vi "Replicate Graph.vi"() -> ()   [LabVIEW 2020, in "Uno.lvclass"]
uses:
  Uno.lvclass
  <vilib>/Analysis/1siggen.llb/Ramp Pattern by Delta.vi
  <vilib>/Analysis/NI_AALBase.lvlib
panel:
  out "Waveform Graph":dbl[][](graph)
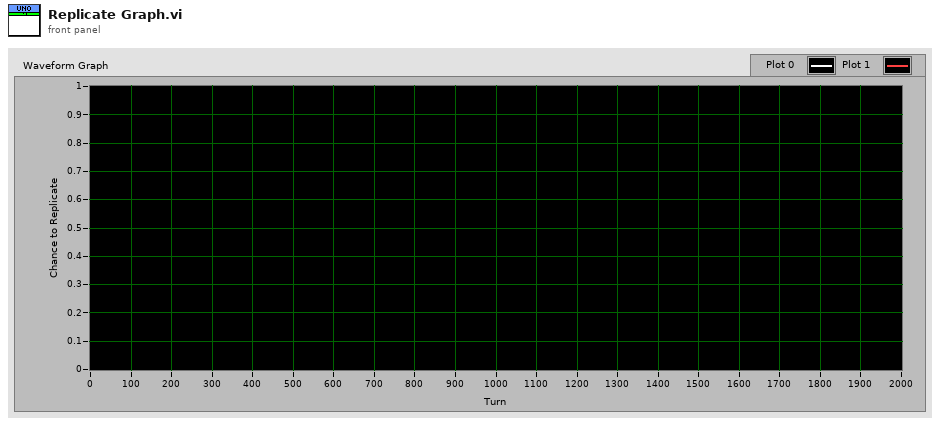
[diagram p1: front panel]
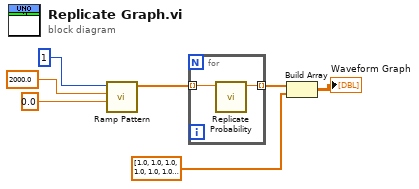
[diagram p0: block diagram]
diagram:
  n1 = call-poly <vilib>:"Ramp Pattern.vi"("start"=0.0, "end"=2000.0, "delta"=1 ("samples")) -> ("Ramp Pattern"=w4:dbl[])  [unwired: 6 in, 2 out]
  n2 = for {
    tunnel: w4 -> [w9] mode=indexing
    tunnel: [w8] -> w3 mode=indexing
    n3 = call "Replicate Probability.vi"("Round in"=w9) -> ("t"=w8:dbl)  [unwired: 10 in]
  }
  n4 = Build Array(w3, dbl[] [1.0, 1.0, 1.0, 1.0, 1.0, 1.0, 1.0, 1.0, 1.0, 1.0, 1.0, 1.0, 1.0, 1.0, 1.0, 1.0, 1.0, 1.0, 1.0, 1.0, 1.0, 1.0, 1.0, 1.0, 1.0, 1.0, 1.0, 1.0, 1.0, 1.0, 1.0, 1.0, 1.0, 1.0, 1.0, 1.0, 1.0, 1.0, 1.0, 1.0, 1.0, 1.0, 1.0, 1.0, 1.0, 1.0, 1.0, 1.0, 1.0, 1.0, 1.0, 1.0, 1.0, 1.0, 1.0, 1.0, 1.0, 1.0, 1.0, 1.0, 1.0, 1.0, 1.0, 1.0, 1.0, 1.0, 1.0, 1.0, 1.0, 1.0, 1.0, 1.0, 1.0, 1.0, 1.0, 1.0, 1.0, 1.0, 1.0, 1.0, 1.0, 1.0, 1.0, 1.0, 1.0, 1.0, 1.0, 1.0, 1.0, 1.0, 1.0, 1.0, 1.0, 1.0, 1.0, 1.0, 1.0, 1.0, 1.0, 1.0, 1.0, 1.0, 1.0, 1.0, 1.0, 1.0, 1.0, 1.0, 1.0, 1.0, 1.0, 1.0, 1.0, 1.0, 1.0, 1.0, 1.0, 1.0, 1.0, 1.0, 1.0, 1.0, 1.0, 1.0, 1.0, 1.0, 1.0, 1.0, 1.0, 1.0, 1.0, 1.0, 1.0, 1.0, 1.0, 1.0, 1.0, 1.0, 1.0, 1.0, 1.0, 1.0, 1.0, 1.0, 1.0, 1.0, 1.0, 1.0, 1.0, 1.0, 1.0, 1.0, 1.0, 1.0, 1.0, 1.0, 1.0, 1.0, 1.0, 1.0, 1.0, 1.0, 1.0, 1.0, 1.0, 1.0, 1.0, 1.0, 1.0, 1.0, 1.0, 1.0, 1.0, 1.0, 1.0, 1.0, 1.0, 1.0, 1.0, 1.0, 1.0, 1.0, 1.0, 1.0, 1.0, 1.0, 1.0, 1.0, 1.0, 1.0, 1.0, 1.0, 1.0, 1.0, 1.0, 1.0, 1.0, 1.0, 1.0, 1.0, 1.0, 1.0, 1.0, 1.0, 1.0, 1.0, 1.0, 1.0, 1.0, 1.0, 1.0, 1.0, 1.0, 1.0, 1.0, 1.0, 1.0, 1.0, 1.0, 1.0, 1.0, 1.0, 1.0, 1.0, 1.0, 1.0, 1.0, 1.0, 1.0, 1.0, 1.0, 1.0, 1.0, 1.0, 1.0, 1.0, 1.0, 1.0, 1.0, 1.0, 1.0, 1.0, 1.0, 1.0, 1.0, 1.0, 1.0, 1.0, 1.0, 1.0, 1.0, 1.0, 1.0, 1.0, 1.0, 1.0, 1.0, 1.0, 1.0, 1.0, 1.0, 1.0, 1.0, 1.0, 1.0, 1.0, 1.0, 1.0, 1.0, 1.0, 1.0, 1.0, 1.0, 1.0, 1.0, 1.0, 1.0, 1.0, 1.0, 1.0, 1.0, 1.0, 1.0, 1.0, 1.0, 1.0, 1.0, 1.0, 1.0, 1.0, 1.0, 1.0, 1.0, 1.0, 1.0, 1.0, 1.0, 1.0, 1.0, 1.0, 1.0, 1.0, 1.0, 1.0, 1.0, 1.0, 1.0, 1.0, 1.0, 1.0, 1.0, 1.0, 1.0, 1.0, 1.0, 1.0, 1.0, 1.0, 1.0, 1.0, 1.0, 1.0, 1.0, 1.0, 1.0, 1.0, 1.0, 1.0, 1.0, 1.0, 1.0, 1.0, 1.0, 1.0, 1.0, 1.0, 1.0, 1.0, 1.0, 1.0, 1.0, 1.0, 1.0, 1.0, 1.0, 1.0, 1.0, 1.0, 1.0, 1.0, 1.0, 1.0, 1.0, 1.0, 1.0, 1.0, 1.0, 1.0, 1.0, 1.0, 1.0, 1.0, 1.0, 1.0, 1.0, 1.0, 1.0, 1.0, 1.0, 1.0, 1.0, 1.0, 1.0, 1.0, 1.0, 1.0, 1.0, 1.0, 1.0, 1.0, 1.0, 1.0, 1.0, 1.0, 1.0, 1.0, 1.0, 1.0, 1.0, 1.0, 1.0, 1.0, 1.0, 1.0, 1.0, 1.0, 1.0, 1.0, 1.0, 1.0, 1.0, 1.0, 1.0, 1.0, 1.0, 1.0, 1.0, 1.0, 1.0, 1.0, 1.0, 1.0, 1.0, 1.0, 1.0, 1.0, 1.0, 1.0, 1.0, 1.0, 1.0, 1.0, 1.0, 1.0, 1.0, 1.0, 1.0, 1.0, 1.0, 1.0, 1.0, 1.0, 1.0, 1.0, 1.0, 1.0, 1.0, 1.0, 1.0, 1.0, 1.0, 1.0, 1.0, 1.0, 1.0, 1.0, 1.0, 1.0, 1.0, 1.0, 1.0, 1.0, 1.0, 1.0, 1.0, 1.0, 1.0, 1.0, 1.0, 1.0, 1.0, 1.0, 1.0, 1.0, 1.0, 1.0, 1.0, 1.0, 1.0, 1.0, 1.0, 1.0, 1.0, 1.0, 1.0, 1.0, 1.0, 1.0, 1.0, 1.0, 1.0, 1.0, 1.0, 1.0, 1.0, 1.0, 1.0, 1.0, 1.0, 1.0, 1.0, 1.0, 1.0, 1.0, 1.0, 1.0, 1.0, 1.0, 1.0, 1.0, 1.0, 1.0, 1.0, 1.0, 1.0, 1.0, 1.0, 1.0, 1.0, 1.0, 1.0, 1.0, 1.0, 1.0, 1.0, 1.0, 1.0, 1.0, 1.0, 1.0, 1.0, 1.0, 1.0, 1.0, 1.0, 1.0, 1.0, 1.0, 1.0, 1.0, 1.0, 1.0, 1.0, 1.0, 1.0, 1.0, 1.0, 1.0, 1.0, 1.0, 1.0, 1.0, 1.0, 1.0, 1.0, 1.0, 1.0, 1.0, 1.0, 1.0, 1.0, 1.0, 1.0, 1.0, 1.0, 1.0, 1.0, 1.0, 1.0, 1.0, 1.0, 1.0, 1.0, 1.0, 1.0, 1.0, 1.0, 1.0, 1.0, 1.0, 1.0, 1.0, 1.0, 1.0, 1.0, 1.0, 1.0, 1.0, 1.0, 1.0, 1.0, 1.0, 1.0, 1.0, 1.0, 1.0, 1.0, 1.0, 1.0, 1.0, 1.0, 1.0, 1.0, 1.0, 1.0, 1.0, 1.0, 1.0, 1.0, 1.0, 1.0, 0.2, 0.2, 0.2, 0.2, 0.2, 0.2, 0.2, 0.2, 0.2, 0.2, 0.2, 0.2, 0.2, 0.2, 0.2, 0.2, 0.2, 0.2, 0.2, 0.2, 0.2, 0.2, 0.2, 0.2, 0.2, 0.2, 0.2, 0.2, 0.2, 0.2, 0.2, 0.2, 0.2, 0.2, 0.2, 0.2, 0.2, 0.2, 0.2, 0.2, 0.9, 0.9, 0.9, 0.9, 0.9, 0.9, 0.9, 0.9, 0.9, 0.9, 0.9, 0.9, 0.9, 0.9, 0.9, 0.9, 0.9, 0.9, 0.9, 0.9, 0.9, 0.9, 0.9, 0.9, 0.9, 0.9, 0.9, 0.9, 0.9, 0.9, 0.9, 0.9, 0.9, 0.9, 0.9, 0.9, 0.9, 0.9, 0.9, 0.9, 0.9, 0.9, 0.9, 0.9, 0.9, 0.9, 0.9, 0.9, 0.9, 0.9, 0.9, 0.9, 0.9, 0.9, 0.9, 0.9, 0.9, 0.9, 0.9, 0.9, 0.9, 0.9, 0.9, 0.9, 0.9, 0.9, 0.9, 0.9, 0.9, 0.9, 0.9, 0.9, 0.9, 0.9, 0.9, 0.9, 0.9, 0.9, 0.9, 0.9, 0.9, 0.9, 0.9, 0.9, 0.9, 0.9, 0.9, 0.9, 0.9, 0.9, 0.9, 0.9, 0.9, 0.9, 0.9, 0.9, 0.9, 0.9, 0.9, 0.9, 0.9, 0.9, 0.9, 0.9, 0.9, 0.9, 0.9, 0.9, 0.9, 0.9, 0.9, 0.9, 0.9, 0.9, 0.9, 0.9, 0.9, 0.9, 0.9, 0.9, 0.9, 0.9, 0.9, 0.9, 0.9, 0.9, 0.9, 0.9, 0.9, 0.9, 0.9, 0.9, 0.9, 0.9, 0.9, 0.9, 0.9, 0.9, 0.9, 0.9, 0.9, 0.9, 0.9, 0.9, 0.9, 0.9, 0.9, 0.9, 0.9, 0.9, 0.9, 0.9, 0.9, 0.9, 0.9, 0.9, 0.9, 0.9, 0.9, 0.9, 0.1, 0.1, 0.1, 0.1, 0.1, 0.1, 0.1, 0.1, 0.1, 0.1, 0.1, 0.1, 0.1, 0.1, 0.1, 0.1, 0.1, 0.1, 0.1, 0.1, 0.1, 0.1, 0.1, 0.1, 0.1, 0.1, 0.1, 0.1, 0.1, 0.1, 0.1, 0.1, 0.1, 0.1, 0.1, 0.1, 0.1, 0.1, 0.1, 0.1, 0.1, 0.1, 0.1, 0.1, 0.1, 0.1, 0.1, 0.1, 0.1, 0.1, 0.7000000000000001, 0.7000000000000001, 0.7000000000000001, 0.7000000000000001, 0.7000000000000001, 0.7000000000000001, 0.7000000000000001, 0.7000000000000001, 0.7000000000000001, 0.7000000000000001, 0.7000000000000001, 0.7000000000000001, 0.7000000000000001, 0.7000000000000001, 0.7000000000000001, 0.7000000000000001, 0.7000000000000001, 0.7000000000000001, 0.7000000000000001, 0.7000000000000001, 0.7000000000000001, 0.7000000000000001, 0.7000000000000001, 0.7000000000000001, 0.7000000000000001, 0.7000000000000001, 0.7000000000000001, 0.7000000000000001, 0.7000000000000001, 0.7000000000000001, 0.7000000000000001, 0.7000000000000001, 0.7000000000000001, 0.7000000000000001, 0.7000000000000001, 0.7000000000000001, 0.7000000000000001, 0.7000000000000001, 0.7000000000000001, 0.7000000000000001, 0.7000000000000001, 0.7000000000000001, 0.7000000000000001, 0.7000000000000001, 0.7000000000000001, 0.7000000000000001, 0.7000000000000001, 0.7000000000000001, 0.7000000000000001, 0.7000000000000001, 0.7000000000000001, 0.7000000000000001, 0.7000000000000001, 0.7000000000000001, 0.7000000000000001, 0.7000000000000001, 0.7000000000000001, 0.7000000000000001, 0.7000000000000001, 0.7000000000000001, 0.7000000000000001, 0.7000000000000001, 0.7000000000000001, 0.7000000000000001, 0.7000000000000001, 0.7000000000000001, 0.7000000000000001, 0.7000000000000001, 0.7000000000000001, 0.7000000000000001, 0.7000000000000001, 0.7000000000000001, 0.7000000000000001, 0.7000000000000001, 0.7000000000000001, 0.7000000000000001, 0.7000000000000001, 0.7000000000000001, 0.7000000000000001, 0.7000000000000001, 0.7000000000000001, 0.7000000000000001, 0.7000000000000001, 0.7000000000000001, 0.7000000000000001, 0.7000000000000001, 0.7000000000000001, 0.7000000000000001, 0.7000000000000001, 0.7000000000000001, 0.7000000000000001, 0.7000000000000001, 0.7000000000000001, 0.7000000000000001, 0.7000000000000001, 0.7000000000000001, 0.7000000000000001, 0.7000000000000001, 0.7000000000000001, 0.7000000000000001, 0.7000000000000001, 0.7000000000000001, 0.7000000000000001, 0.7000000000000001, 0.7000000000000001, 0.7000000000000001, 0.7000000000000001, 0.7000000000000001, 0.7000000000000001, 0.7000000000000001, 0.7000000000000001, 0.7000000000000001, 0.7000000000000001, 0.7000000000000001, 0.7000000000000001, 0.7000000000000001, 0.7000000000000001, 0.7000000000000001, 0.7000000000000001, 0.7000000000000001, 0.7000000000000001, 0.7000000000000001, 0.7000000000000001, 0.7000000000000001, 0.7000000000000001, 0.7000000000000001, 0.7000000000000001, 0.7000000000000001, 0.7000000000000001, 0.7000000000000001, 0.7000000000000001, 0.7000000000000001, 0.7000000000000001, 0.7000000000000001, 0.7000000000000001, 0.7000000000000001, 0.7000000000000001, 0.7000000000000001, 0.7000000000000001, 0.7000000000000001, 0.7000000000000001, 0.7000000000000001, 0.7000000000000001, 0.7000000000000001, 0.7000000000000001, 0.7000000000000001, 0.7000000000000001, 0.7000000000000001, 0.7000000000000001, 0.7000000000000001, 0.02, 0.02, 0.02, 0.02, 0.02, 0.02, 0.02, 0.02, 0.02, 0.02, 0.02, 0.02, 0.02, 0.02, 0.02, 0.02, 0.02, 0.02, 0.02, 0.02, 0.02, 0.02, 0.02, 0.02, 0.02, 0.02, 0.02, 0.02, 0.02, 0.02, 0.02, 0.02, 0.02, 0.02, 0.02, 0.02, 0.02, 0.02, 0.02, 0.02, 0.02, 0.02, 0.02, 0.02, 0.02, 0.02, 0.02, 0.02, 0.02, 0.02, 0.02, 0.02, 0.02, 0.02, 0.02, 0.02, 0.02, 0.02, 0.02, 0.02, 0.02, 0.02, 0.02, 0.02, 0.02, 0.02, 0.02, 0.02, 0.02, 0.02, 0.02, 0.02, 0.02, 0.02, 0.02, 0.02, 0.02, 0.02, 0.02, 0.02, 0.02, 0.02, 0.02, 0.02, 0.02, 0.02, 0.02, 0.02, 0.02, 0.02, 0.02, 0.02, 0.02, 0.02, 0.02, 0.02, 0.02, 0.02, 0.02, 0.02, 0.09, 0.09, 0.09, 0.09, 0.09, 0.09, 0.09, 0.09, 0.09, 0.09, 0.09, 0.09, 0.09, 0.09, 0.09, 0.09, 0.09, 0.09, 0.09, 0.09, 0.09, 0.09, 0.09, 0.09, 0.09, 0.09, 0.09, 0.09, 0.09, 0.09, 0.09, 0.09, 0.09, 0.09, 0.09, 0.09, 0.09, 0.09, 0.09, 0.09, 0.09, 0.09, 0.09, 0.09, 0.09, 0.09, 0.09, 0.09, 0.09, 0.09, 0.09, 0.09, 0.09, 0.09, 0.09, 0.09, 0.09, 0.09, 0.09, 0.09, 0.09, 0.09, 0.09, 0.09, 0.09, 0.09, 0.09, 0.09, 0.09, 0.09, 0.09, 0.09, 0.09, 0.09, 0.09, 0.09, 0.09, 0.09, 0.09, 0.09, 0.09, 0.09, 0.09, 0.09, 0.09, 0.09, 0.09, 0.09, 0.09, 0.09, 0.09, 0.09, 0.09, 0.09, 0.09, 0.09, 0.09, 0.09, 0.09, 0.09, 0.05, 0.05, 0.05, 0.05, 0.05, 0.05, 0.05, 0.05, 0.05, 0.05, 0.05, 0.05, 0.05, 0.05, 0.05, 0.05, 0.05, 0.05, 0.05, 0.05, 0.05, 0.05, 0.05, 0.05, 0.05, 0.05, 0.05, 0.05, 0.05, 0.05, 0.05, 0.05, 0.05, 0.05, 0.05, 0.05, 0.05, 0.05, 0.05, 0.05, 0.05, 0.05, 0.05, 0.05, 0.05, 0.05, 0.05, 0.05, 0.05, 0.05, 0.05, 0.05, 0.05, 0.05, 0.05, 0.05, 0.05, 0.05, 0.05, 0.05, 0.05, 0.05, 0.05, 0.05, 0.05, 0.05, 0.05, 0.05, 0.05, 0.05, 0.05, 0.05, 0.05, 0.05, 0.05, 0.05, 0.05, 0.05, 0.05, 0.05, 0.05, 0.05, 0.05, 0.05, 0.05, 0.05, 0.05, 0.05, 0.05, 0.05, 0.05, 0.05, 0.05, 0.05, 0.05, 0.05, 0.05, 0.05, 0.05, 0.05, 0.03, 0.03, 0.03, 0.03, 0.03, 0.03, 0.03, 0.03, 0.03, 0.03, 0.03, 0.03, 0.03, 0.03, 0.03, 0.03, 0.03, 0.03, 0.03, 0.03, 0.03, 0.03, 0.03, 0.03, 0.03, 0.03, 0.03, 0.03, 0.03, 0.03, 0.03, 0.03, 0.03, 0.03, 0.03, 0.03, 0.03, 0.03, 0.03, 0.03, 0.03, 0.03, 0.03, 0.03, 0.03, 0.03, 0.03, 0.03, 0.03, 0.03, 0.03, 0.03, 0.03, 0.03, 0.03, 0.03, 0.03, 0.03, 0.03, 0.03, 0.03, 0.03, 0.03, 0.03, 0.03, 0.03, 0.03, 0.03, 0.03, 0.03, 0.03, 0.03, 0.03, 0.03, 0.03, 0.03, 0.03, 0.03, 0.03, 0.03, 0.03, 0.03, 0.03, 0.03, 0.03, 0.03, 0.03, 0.03, 0.03, 0.03, 0.03, 0.03, 0.03, 0.03, 0.03, 0.03, 0.03, 0.03, 0.03, 0.03, 0.010000000000000002, 0.010000000000000002, 0.010000000000000002, 0.010000000000000002, 0.010000000000000002, 0.010000000000000002, 0.010000000000000002, 0.010000000000000002, 0.010000000000000002, 0.010000000000000002, 0.010000000000000002, 0.010000000000000002, 0.010000000000000002, 0.010000000000000002, 0.010000000000000002, 0.010000000000000002, 0.010000000000000002, 0.010000000000000002, 0.010000000000000002, 0.010000000000000002, 0.010000000000000002, 0.010000000000000002, 0.010000000000000002, 0.010000000000000002, 0.010000000000000002, 0.010000000000000002, 0.010000000000000002, 0.010000000000000002, 0.010000000000000002, 0.010000000000000002, 0.010000000000000002, 0.010000000000000002, 0.010000000000000002, 0.010000000000000002, 0.010000000000000002, 0.010000000000000002, 0.010000000000000002, 0.010000000000000002, 0.010000000000000002, 0.010000000000000002, 0.010000000000000002, 0.010000000000000002, 0.010000000000000002, 0.010000000000000002, 0.010000000000000002, 0.010000000000000002, 0.010000000000000002, 0.010000000000000002, 0.010000000000000002, 0.010000000000000002, 0.010000000000000002, 0.010000000000000002, 0.010000000000000002, 0.010000000000000002, 0.010000000000000002, 0.010000000000000002, 0.010000000000000002, 0.010000000000000002, 0.010000000000000002, 0.010000000000000002, 0.010000000000000002, 0.010000000000000002, 0.010000000000000002, 0.010000000000000002, 0.010000000000000002, 0.010000000000000002, 0.010000000000000002, 0.010000000000000002, 0.010000000000000002, 0.010000000000000002, 0.010000000000000002, 0.010000000000000002, 0.010000000000000002, 0.010000000000000002, 0.010000000000000002, 0.010000000000000002, 0.010000000000000002, 0.010000000000000002, 0.010000000000000002, 0.010000000000000002, 0.010000000000000002, 0.010000000000000002, 0.010000000000000002, 0.010000000000000002, 0.010000000000000002, 0.010000000000000002, 0.010000000000000002, 0.010000000000000002, 0.010000000000000002, 0.010000000000000002, 0.010000000000000002, 0.010000000000000002, 0.010000000000000002, 0.010000000000000002, 0.010000000000000002, 0.010000000000000002, 0.010000000000000002, 0.010000000000000002, 0.010000000000000002, 0.010000000000000002, 0.010000000000000002, 0.010000000000000002, 0.010000000000000002, 0.010000000000000002, 0.010000000000000002, 0.010000000000000002, 0.010000000000000002, 0.010000000000000002, 0.010000000000000002, 0.010000000000000002, 0.010000000000000002, 0.010000000000000002, 0.010000000000000002, 0.010000000000000002, 0.010000000000000002, 0.010000000000000002, 0.010000000000000002, 0.010000000000000002, 0.010000000000000002, 0.010000000000000002, 0.010000000000000002, 0.010000000000000002, 0.010000000000000002, 0.010000000000000002, 0.010000000000000002, 0.010000000000000002, 0.010000000000000002, 0.010000000000000002, 0.010000000000000002, 0.010000000000000002, 0.010000000000000002, 0.010000000000000002, 0.010000000000000002, 0.010000000000000002, 0.010000000000000002, 0.010000000000000002, 0.010000000000000002, 0.010000000000000002, 0.010000000000000002, 0.010000000000000002, 0.010000000000000002, 0.010000000000000002, 0.010000000000000002, 0.010000000000000002, 0.010000000000000002, 0.010000000000000002, 0.010000000000000002, 0.010000000000000002, 0.010000000000000002, 0.010000000000000002, 0.010000000000000002, 0.010000000000000002, 0.010000000000000002, 0.010000000000000002, 0.010000000000000002, 0.010000000000000002, 0.010000000000000002, 0.010000000000000002, 0.010000000000000002, 0.010000000000000002, 0.010000000000000002, 0.010000000000000002, 0.010000000000000002, 0.010000000000000002, 0.010000000000000002, 0.010000000000000002, 0.010000000000000002, 0.010000000000000002, 0.010000000000000002, 0.010000000000000002, 0.010000000000000002, 0.010000000000000002, 0.010000000000000002, 0.010000000000000002, 0.010000000000000002, 0.010000000000000002, 0.010000000000000002, 0.010000000000000002, 0.010000000000000002, 0.010000000000000002, 0.010000000000000002, 0.010000000000000002, 0.010000000000000002, 0.010000000000000002, 0.010000000000000002, 0.010000000000000002, 0.010000000000000002, 0.010000000000000002, 0.010000000000000002, 0.010000000000000002, 0.010000000000000002, 0.010000000000000002, 0.010000000000000002, 0.010000000000000002, 0.010000000000000002, 0.010000000000000002, 0.010000000000000002, 0.010000000000000002, 0.010000000000000002, 0.010000000000000002, 0.008, 0.008, 0.008, 0.008, 0.008, 0.008, 0.008, 0.008, 0.008, 0.008, 0.008, 0.008, 0.008, 0.008, 0.008, 0.008, 0.008, 0.008, 0.008, 0.008, 0.008, 0.008, 0.008, 0.008, 0.008, 0.008, 0.008, 0.008, 0.008, 0.008, 0.008, 0.008, 0.008, 0.008, 0.008, 0.008, 0.008, 0.008, 0.008, 0.008, 0.008, 0.008, 0.008, 0.008, 0.008, 0.008, 0.008, 0.008, 0.008, 0.008, 0.008, 0.008, 0.008, 0.008, 0.008, 0.008, 0.008, 0.008, 0.008, 0.008, 0.008, 0.008, 0.008, 0.008, 0.008, 0.008, 0.008, 0.008, 0.008, 0.008, 0.008, 0.008, 0.008, 0.008, 0.008, 0.008, 0.008, 0.008, 0.008, 0.008, 0.008, 0.008, 0.008, 0.008, 0.008, 0.008, 0.008, 0.008, 0.008, 0.008, 0.008, 0.008, 0.008, 0.008, 0.008, 0.008, 0.008, 0.008, 0.008, 0.008, 0.008, 0.008, 0.008, 0.008, 0.008, 0.008, 0.008, 0.008, 0.008, 0.008, 0.008, 0.008, 0.008, 0.008, 0.008, 0.008, 0.008, 0.008, 0.008, 0.008, 0.008, 0.008, 0.008, 0.008, 0.008, 0.008, 0.008, 0.008, 0.008, 0.008, 0.008, 0.008, 0.008, 0.008, 0.008, 0.008, 0.008, 0.008, 0.008, 0.008, 0.008, 0.008, 0.008, 0.008, 0.008, 0.008, 0.008, 0.008, 0.008, 0.008, 0.008, 0.008, 0.008, 0.008, 0.008, 0.008, 0.008, 0.008, 0.008, 0.008, 0.008, 0.008, 0.008, 0.008, 0.008, 0.008, 0.008, 0.008, 0.008, 0.008, 0.008, 0.008, 0.008, 0.008, 0.008, 0.008, 0.008, 0.008, 0.008, 0.008, 0.008, 0.008, 0.008, 0.008, 0.008, 0.008, 0.008, 0.008, 0.008, 0.008, 0.008, 0.008, 0.008, 0.008, 0.008, 0.008, 0.008, 0.008, 0.008, 0.008, 0.008, 0.008, 0.008, 0.008, 0.008, 0.008, 0.008, 0.008, 0.008, 0.008, 0.008, 0.008, 0.008, 0.008, 0.008, 0.008, 0.008, 0.008, 0.008, 0.008, 0.008, 0.008, 0.008, 0.008, 0.008, 0.008, 0.008, 0.008, 0.008, 0.008, 0.008, 0.008, 0.008, 0.008, 0.008, 0.008, 0.008, 0.008, 0.008, 0.008, 0.008, 0.008, 0.008, 0.008, 0.008, 0.008, 0.008, 0.008, 0.008, 0.008, 0.008, 0.008, 0.008, 0.008, 0.008, 0.008, 0.008, 0.008, 0.008, 0.008, 0.008, 0.008, 0.008, 0.008, 0.008, 0.008, 0.008, 0.008, 0.008, 0.008, 0.008, 0.008, 0.008, 0.008, 0.008, 0.008, 0.008, 0.008, 0.008, 0.008, 0.008, 0.008, 0.008, 0.008, 0.008, 0.008, 0.008, 0.008, 0.008, 0.008, 0.008, 0.008, 0.008, 0.008, 0.008, 0.008, 0.008, 0.008, 0.008, 0.008, 0.008, 0.008, 0.008, 0.008, 0.008, 0.008, 0.008, 0.008, 0.008, 0.008, 0.008, 0.008, 0.008, 0.008, 0.008, 0.008, 0.008, 0.008, 0.008, 0.008, 0.008, 0.008, 0.008, 0.008, 0.008, 0.008, 0.008, 0.008, 0.008, 0.008, 0.008, 0.008, 0.008, 0.008, 0.008, 0.008, 0.008, 0.008, 0.008, 0.008, 0.008, 0.008, 0.008, 0.008, 0.008, 0.008, 0.008, 0.008, 0.008, 0.008, 0.008, 0.008, 0.008, 0.008, 0.008, 0.008, 0.008, 0.008, 0.008, 0.008, 0.008, 0.008, 0.008, 0.008, 0.008, 0.008, 0.008, 0.008, 0.008, 0.008, 0.008, 0.008, 0.008, 0.008, 0.008, 0.008, 0.008, 0.008, 0.008, 0.008, 0.008, 0.008, 0.008, 0.008, 0.008, 0.008, 0.008, 0.008, 0.008, 0.008, 0.008, 0.008, 0.008, 0.008, 0.008, 0.008, 0.008, 0.008, 0.008, 0.008] ("Waveform Graph")) -> (→"Waveform Graph":dbl[][])
